vi "Get Object Item by Path.vi"(7 "Item Path":string, 8 "error in (no error)":errorcluster, 10 "Object Offset":i32, 11 "JSON":string) -> (0 "error out":errorcluster, 1 "<JSON>":string caption="JSON substring", 2 "Item Offset (-1 if not found)":i32, 3 "Found":bool)   [LabVIEW 2013, in "JSONtext.lvlib"]
uses:
  JSONtext.lvlib
  support/JSONtext support.lvlib
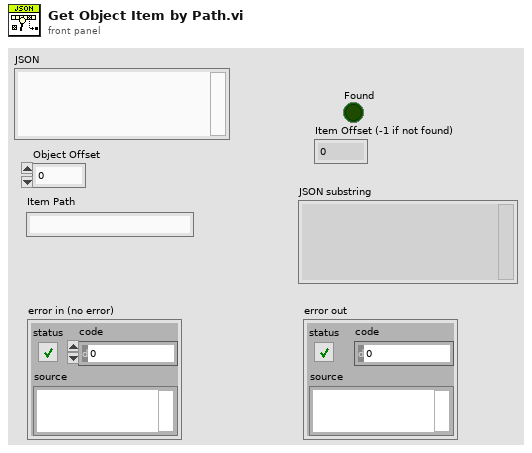
[diagram p1: front panel]
types:
  T1 = typedef "JSONtext.lvlib/Parsing State.ctl" = enum16{"Parser Error", "Object", "Array", "String", "Number/Other", "Leading Whitespace", "Object end", "Array end", "Value end"}
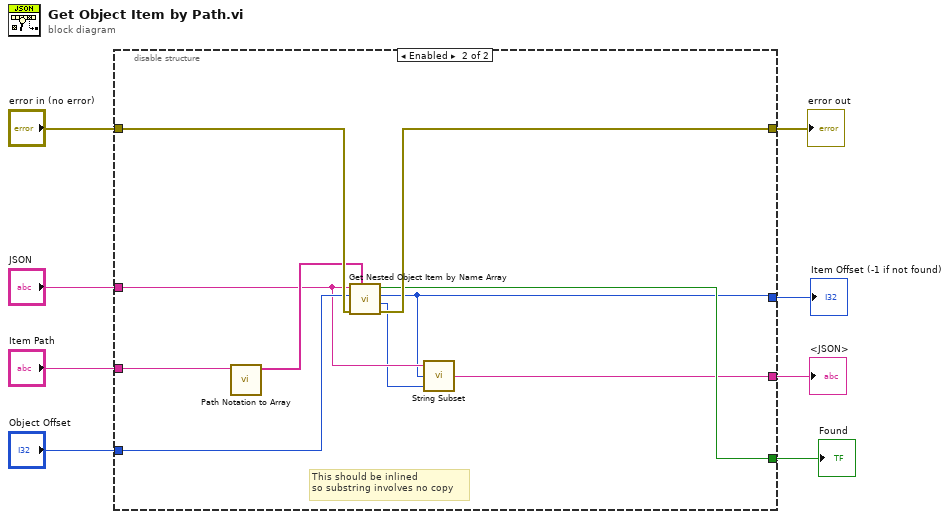
[diagram p0: block diagram]
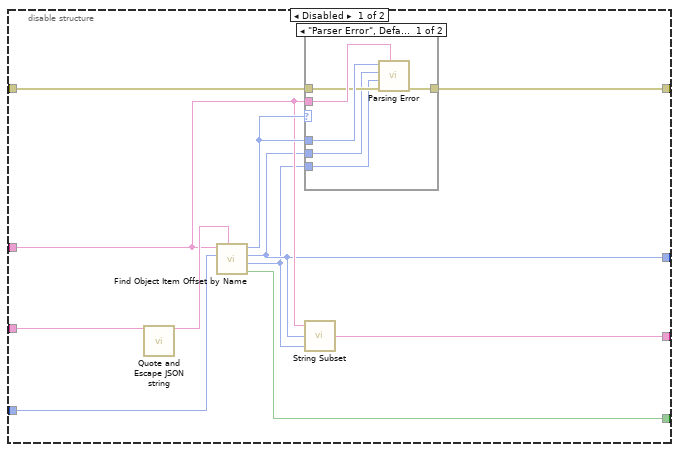
[diagram p2: hidden frame]
diagram:
  n1 = disable-structure shown="Enabled" {
    disable-tunnel: [w19 w27] -> w8
    disable-tunnel: "Item Path" -> [w18 w33]
    disable-tunnel: [w17 w34] -> w6
    disable-tunnel: "Object Offset" -> [w16 w32]
    disable-tunnel: "error in (no error)" -> [w13 w36]
    disable-tunnel: [w12 w35] -> w3
    disable-tunnel: "JSON" -> [w11 w30]
    disable-tunnel: [w10 w28] -> w1
    frame Disabled {
      n2 = call "Quote and Escape JSON string.vi"("Plain Text"=w18) -> ("<JSON>"=w14:string)  [unwired: 10 in]
      n3 = call "Find Object Item Offset by Name.vi"("Item Name <JSON>"=w14, "Object Offset"=w16, "JSON"=w11) -> ("Found"=w17:bool, "Offset past Item (or past last Item, if not found)"=w9:i32, "Item Offset (-1 if not found)"=w10:i32, "State"=w15:T1)  [unwired: 4 in, 1 out]
      n4 = case shown="\"Parser Error\", Default" w15 {
        tunnel: w15 -> [w25 _]
        tunnel: w11 -> [w24 _]
        tunnel: w13 -> [w23 w26]
        tunnel: [w22 w26] -> w12
        tunnel: w10 -> [w21 _]
        tunnel: w9 -> [w20 _]
        frame "Parser Error", Default {
          n5 = call "Parsing Error.vi"("JSON"=w24, "error in (no error)"=w23, "Offset past match"=w20, "Value start"=w21, "State"=w25) -> ("error out"=w22:errorcluster)  [unwired: 6 in]
        }
        frame "Value end" {
        }
      }
      n6 = call "String Subset.vi"("Offset past End"=w9, "Start offset"=w10, "JSON"=w11) -> ("substring"=w19:string)  [unwired: 2 in]
    }
    frame Enabled {
      # "This should be inlined\nso substring involves no copy"
      n7 = call "Path Notation to Array.vi"("Item Path"=w33) -> ("Nested Item Names"=w31:string[])  [unwired: 10 in]
      n8 = call "Get Nested Object Item by Name Array.vi"("Item Path (as array of names)"=w31, "error in (no error)"=w36, "Object Offset"=w32, "JSON"=w30) -> ("error out"=w35:errorcluster, "Offset past Item (or past last Item, if not found)"=w29:i32, "Item Offset (-1 if not found)"=w28:i32, "Found"=w34:bool)  [unwired: 4 in]
      n9 = call "String Subset.vi"("Offset past End"=w29, "Start offset"=w28, "JSON"=w30) -> ("substring"=w27:string)  [unwired: 2 in]
    }
  }
  "<JSON>" <- w8
  "Found" <- w6
  "Item Offset (-1 if not found)" <- w1
  "error out" <- w3
